vi "Draw Circle.vi"(0 "GetOverContent IN":refnum<k24>, 7 "Center":cluster{"x":sgl, "y":sgl}, 11 "error in (no error)":errorcluster, 12 "r":sgl, 13 "Color Box":u32(colorbox)) -> (4 "GetOverContent OUT":refnum<k24>, 15 "error out":errorcluster)   [LabVIEW 2019, in "Exaprom PDF.lvlib"]
doc: "Version 1.0\nDeveloped by Jean-Marc Simard\nCopyright © 2010, Exaprom Inc.\nAll rights reserved.\nLicense: BSD\n\nWith iTextSharp 4.1.6 (http://itextsharp.sourceforge.net)\nunder Mozilla Public License Version 1.1\n(http://www.mozilla.org/MPL/MPL-1.1.html)"
uses:
  C:/work/niobrara_lv/labview pdf writer fixing/DLL/itextsharp.dll
  DLL/itextsharp.dll
  Controls/General Controls/CB SetColor.ctl
  Exaprom PDF.lvlib
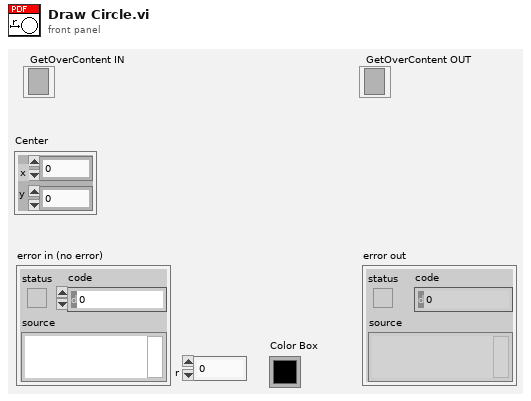
[diagram p1: front panel]
types:
  T1 = typedef "Exaprom PDF.lvlib/CB SetColor.ctl" = enum16{"Fill", "Stroke"}
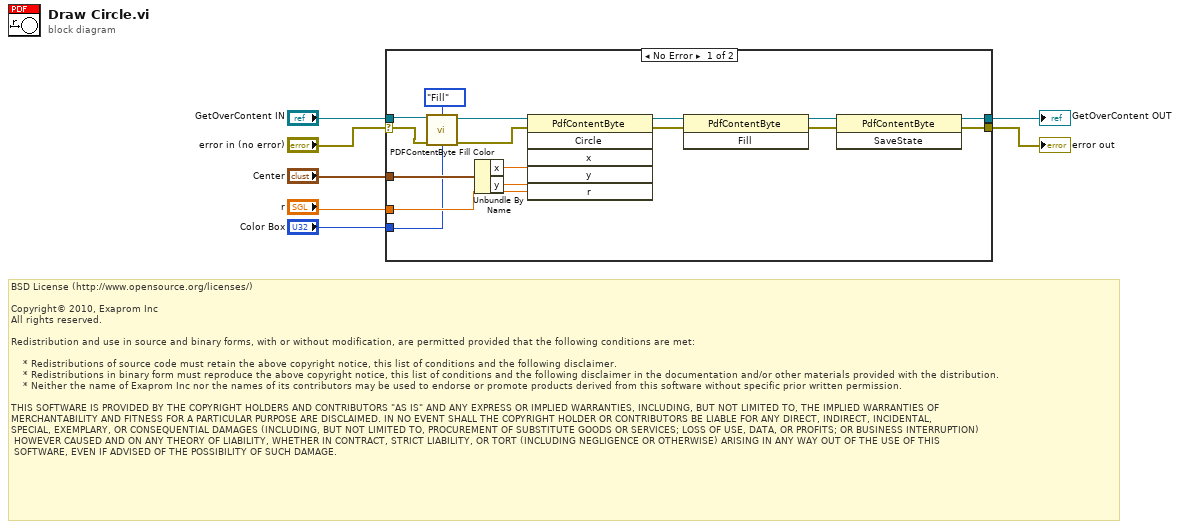
[diagram p0: block diagram]
diagram:
  # "BSD License (http://www.opensource.org/licenses/)\n\nCopyright© 2010, Exaprom Inc\nAll rights reserved.\n\nRedistribution and use in source and binary forms, with or without modification, are permitted provided that the following conditions are met:\n\n    * Redistributions of source code must retain the above copyright notice, this list of conditions and the following disclaimer.\n    * Redistributions in binary form must reproduce the above copyright notice, this list of conditions and the following disclaimer in the documentation and/or other materials provided with the distribution.\n    * Neither the name of Exaprom Inc nor the names of its contributors may be used to endorse or promote products derived from this software without specific prior written permission.\n\nTHIS SOFTWARE IS PROVIDED BY THE COPYRIGHT HOLDERS AND CONTRIBUTORS \"AS IS\" AND ANY EXPRESS OR IMPLIED WARRANTIES, INCLUDING, BUT NOT LIMITED TO, THE IMPLIED WARRANTIES OF \nMERCHANTABILITY AND FITNESS FOR A PARTICULAR PURPOSE ARE DISCLAIMED. IN NO EVENT SHALL THE COPYRIGHT HOLDER OR CONTRIBUTORS BE LIABLE FOR ANY DIRECT, INDIRECT, INCIDENTAL,\nSPECIAL, EXEMPLARY, OR CONSEQUENTIAL DAMAGES (INCLUDING, BUT NOT LIMITED TO, PROCUREMENT OF SUBSTITUTE GOODS OR SERVICES; LOSS OF USE, DATA, OR PROFITS; OR BUSINESS INTERRUPTION)\n HOWEVER CAUSED AND ON ANY THEORY OF LIABILITY, WHETHER IN CONTRACT, STRICT LIABILITY, OR TORT (INCLUDING NEGLIGENCE OR OTHERWISE) ARISING IN ANY WAY OUT OF THE USE OF THIS\n SOFTWARE, EVEN IF ADVISED OF THE POSSIBILITY OF SUCH DAMAGE."
  n1 = case shown="No Error" "error in (no error)" {
    selector: "error in (no error)" -> [w9 w24]
    tunnel: "GetOverContent IN" -> [w12 w25]
    tunnel: [w16 w25] -> w6
    tunnel: "Color Box" -> [w11 _]
    tunnel: [w15 w24] -> w3
    tunnel: "Center" -> [w19 _]
    tunnel: "r" -> [w14 _]
    frame No Error {
      n2 = call "PDFContentByte Fill Color.vi"("PDFContentByte"=w12, "CB SetColor"=CB_SetColor."Fill", "error in (no error)"=w9, "Color Box"=w11) -> ("PDFContentByte duplicate"=w13:refnum<k24>, "error out"=w10:errorcluster)  [unwired: 10 out]
      n3 = Unbundle By Name(w19) -> ("x"=w18:sgl, "y"=w17:sgl)
      n4 = invoke class="PdfContentByte" method="Circle"(reference=w13, error in=w10, "x"=w18, "y"=w17, "r"=w14) -> (reference out=w23:refnum<k24>, error out=w22:errorcluster)  [unwired: 1 in, 4 out]
      n5 = invoke class="PdfContentByte" method="Fill"(reference=w23, error in=w22) -> (reference out=w21:refnum<k24>, error out=w20:errorcluster)  [unwired: 1 in, 1 out]
      n6 = invoke class="PdfContentByte" method="SaveState"(reference=w21, error in=w20) -> (reference out=w16:refnum<k24>, error out=w15:errorcluster)  [unwired: 1 in, 1 out]
    }
    frame Error {
    }
  }
  "GetOverContent OUT" <- w6
  "error out" <- w3
